vi "play_AFMss_integral_trajTrack.vi"() -> ()   [LabVIEW 2017]
uses:
  controls/controlParams_tracktraj.ctl
  <vilib>/userdefined/High Color/nirio_resource_hc.ctl
  <vilib>/Utility/file.llb/Read From Spreadsheet File (DBL).vi
  <vilib>/FPGAPlugInAG/cRIO-9082/niLvFpga_Open_cRIO-9082.vi
  <vilib>/rvi/interface/common/dynamic/niFpgaDynamicAddResources.vi
  <vilib>/FPGAPlugInAG/Dynamic/niLvFpga_Reset_Dynamic.vi
  <vilib>/rvi/interface/common/niFpgaWaitOnOcc.vi
  <vilib>/Utility/error.llb/Error Cluster From Error Code.vi
  <vilib>/rvi/errors/niLvFpgaAdjustHostInterfaceError.vi
  <vilib>/FPGAPlugInAG/Dynamic/niLvFpga_Run_Dynamic.vi
  <vilib>/Utility/file.llb/Write To Spreadsheet File (DBL).vi
  <vilib>/FPGAPlugInAG/Dynamic/niLvFpga_Close_Dynamic.vi
  <vilib>/rvi/interface/nirviOpenFPGA/nirviOpenFPGA.xnode
  FPGA Bitfiles/AFMsssinglematri_FPGATargetSPARTA_AFMsscontrolDela_bcNq5xaO9wQ.lvbitx
  <vilib>/rvi/interface/nirviMethod/nirviMethod.xnode
  <vilib>/rvi/interface/nirviReadWriteControl/nirviReadWriteControl.xnode
  <vilib>/rvi/interface/nirviCloseFPGA/nirviCloseFPGA.xnode
  <vilib>/FPGAPlugInAG/Dynamic/niLvFpga_ConfigureFifo_Dynamic.vi
  <vilib>/rvi/errors/niLvFpgaMergeErrorWithErrorCode.vi
  <vilib>/rvi/interface/Simulation/niFpgaSimulationCallBeginRW.vi
  <vilib>/FPGAPlugInAG/Dynamic/niLvFpga_ReadFifo_Dynamic.vi
  <vilib>/FPGAPlugInAG/Dynamic/niLvFpga_WriteFifo_Dynamic.vi
  NiFpgaLv.dll
panel:
  in  "control_data_path":path=path "C:/Users/arnold/Documents/MATLAB/AFM_SS/data/ref_traj_track.csv"
  out "Actual Depth":u32
  out "YK TO":bool
  out "UK TO":bool
  out "yk":sgl
  out "loop ticks benchmark":sgl
  out "Xd_out(k+1)":sgl[](array[numeric])
  in  "Cluster":T1={"umax"=3.0, "y_ref(k)"=0.0, "Ki"=0.0, "y(k) (from plant)"=0.0, "ND"=0, "NS"=0, "u_Kx_ref(k)"=0.0} {"u_Kx_ref(k)" format="%#_13g"; "Ki" format="%#_13g"; "y_ref(k)" format="%#_13g"; "umax" format="%#_13g"}
  out "Unstable Traj":bool
  out "Control Loop Done":bool
  out "Elements Remaining":u32
  out "Arow10":sgl[](array[numeric])=[0.0, 0.0, 0.0, 0.0, 0.0, 0.0, 0.90156674, 0.0, 0.0]
  out "Arow9":sgl[](array[numeric])=[0.0, 0.0, 0.0, 0.0, 0.0, 0.0, 0.90156674, 0.0, 0.0]
  out "Arow8":sgl[](array[numeric])=[0.0, 0.0, 0.0, 0.0, 0.0, 0.0, 0.90156674, 0.0, 0.0]
  out "elements left":i32=1
  in  "reference traj path":path=path "C:/Users/arnold/Documents/MATLAB/AFM_SS/data/ref_traj_track.csv"
  in  "outputData BOTH":path=path "C:/Users/arnold/Documents/MATLAB/AFM_SS/data/exp01outputBOTH.csv"
  out "x+1":i32
  out "ND":i32
  out "NS":i32
  in  "Tab Control":enum32{"Custom Params", "Loaded Params"}(tab)
  in  "Nbar":dbl=1.253469179440319 format="%#_13g"
  in  "Ki":dbl=0.125346917944 format="%#_13g"
  out "Nbar":dbl=1.253469179440319 format="%#_13g"
  out "Ki":dbl=0.125346917944 format="%#_13g"
  out "ref":dbl format="%#_13g"
  in  "SettleTicks":i32=10
  in  "Stop":bool=TRUE
  out "y iter":i32
  out "u iter":i32
  out "size(s) 5":i32
  out "size(s)":i32
  out "Arow7":sgl[](array[numeric])=[0.0, 0.0, 0.0, 0.0, 0.0, 0.0, 0.90156674, 0.0, 0.0]
  out "Arow6":sgl[](array[numeric])=[0.0, 0.0, 0.0, 0.0, -0.0009308535, 0.009943728, 1.1488396, 0.0, 0.0]
  out "Arow5":sgl[](array[numeric])=[0.0, 0.0, 0.0, 0.0, 0.99437284, 0.09308535, 3.730764, 0.0, 0.0]
  out "Arow4":sgl[](array[numeric])=[0.0, 0.0, -0.16696692, 0.97962993, 29.579603, 1.2871753, 39.36298, 0.0, 0.0]
  out "Arow3":sgl[](array[numeric])=[0.0, 0.0, 0.97962993, 0.16696692, 2.4679432, 0.11174757, 2.9240768, 0.0, 0.0]
  out "K_in 2":sgl[](array[numeric])=[-0.023819132, 0.00010408472, 0.0, 0.0, 0.0, 0.0, 0.0, 0.0, 0.0]
  out "K_in":sgl[](array[numeric])=[-0.023819132, 0.00010408472, 0.0, 0.0, 0.0, 0.0, 0.0, 0.0, 0.0]
  out "Arow2_in":sgl[](array[numeric])=[-0.21879435, 0.97156703, 5.4823804, 0.59487915, 7.8694544, 0.30187303, 8.202156, 0.0, 0.0]
  out "Arow1_in":sgl[](array[numeric])=[0.97156703, 0.21879435, 0.7281903, 0.07828272, 1.117765, 0.037789278, 0.6448556, 0.0, 0.0]
  out "C_in":sgl[](array[numeric])=[-8.076578e-08, -5.6617e-09, 2.3556278e-05, -6.9169624e-07, -0.005420799, 0.00037984832, -0.012524399, 0.0, 0.0]
  out "L_in":sgl[](array[numeric])=[-2254.4756, -17288.861, -3886.0125, -24956.67, -705.887, -3987.6506, -7.2153935, 0.0, 0.0]
  out "Bz_in":sgl[](array[numeric])=[-0.0016434871, -0.020676594, -0.010679029, -0.20639984, -0.030792456, -1.3413852, -0.02736353, 0.0, 0.0]
  in  "Iters":i32=25
  in  "Cont Run (F)":bool=TRUE
  in  "ymax":dbl=4.0 format="%#_13g"
  in  "umax":dbl=1.0 format="%#_13g"
  in  "TsTicks":i32=1600
  # "Manually define Parameters"
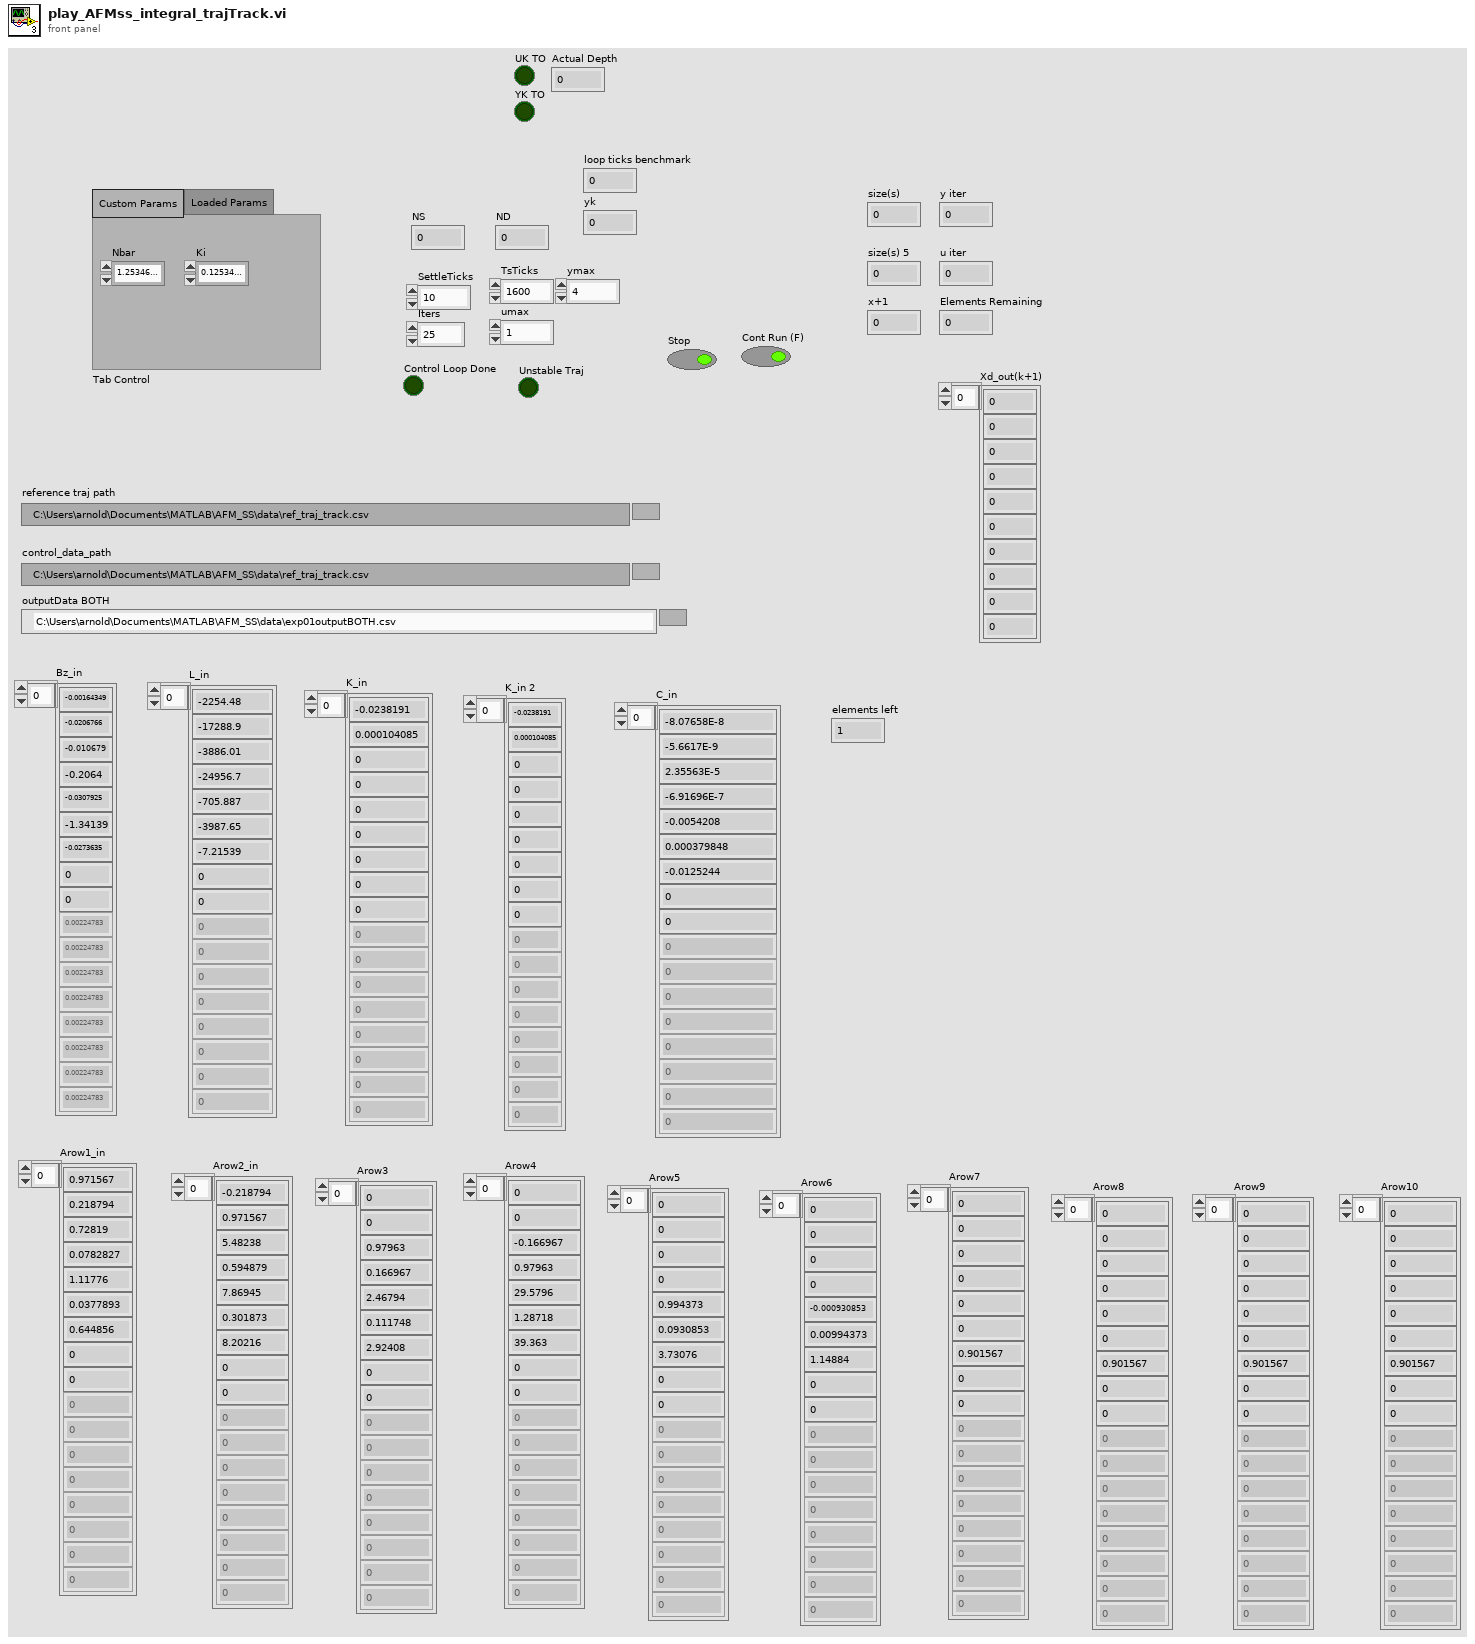
[diagram p1: front panel]
types:
  T1 = typedef "controlParams_tracktraj.ctl" = cluster{"umax":sgl, "y_ref(k)":sgl, "Ki":sgl, "y(k) (from plant)":sgl, "ND":i16, "NS":i16, "u_Kx_ref(k)":sgl}
  T2 = typedef "nirio_resource_hc.ctl" = tag
  T3 = typedef "ControlParams.ctl" = cluster{"NS":i32, "ND":i32, "Nbar":dbl, "Ki":dbl, "ref":dbl}
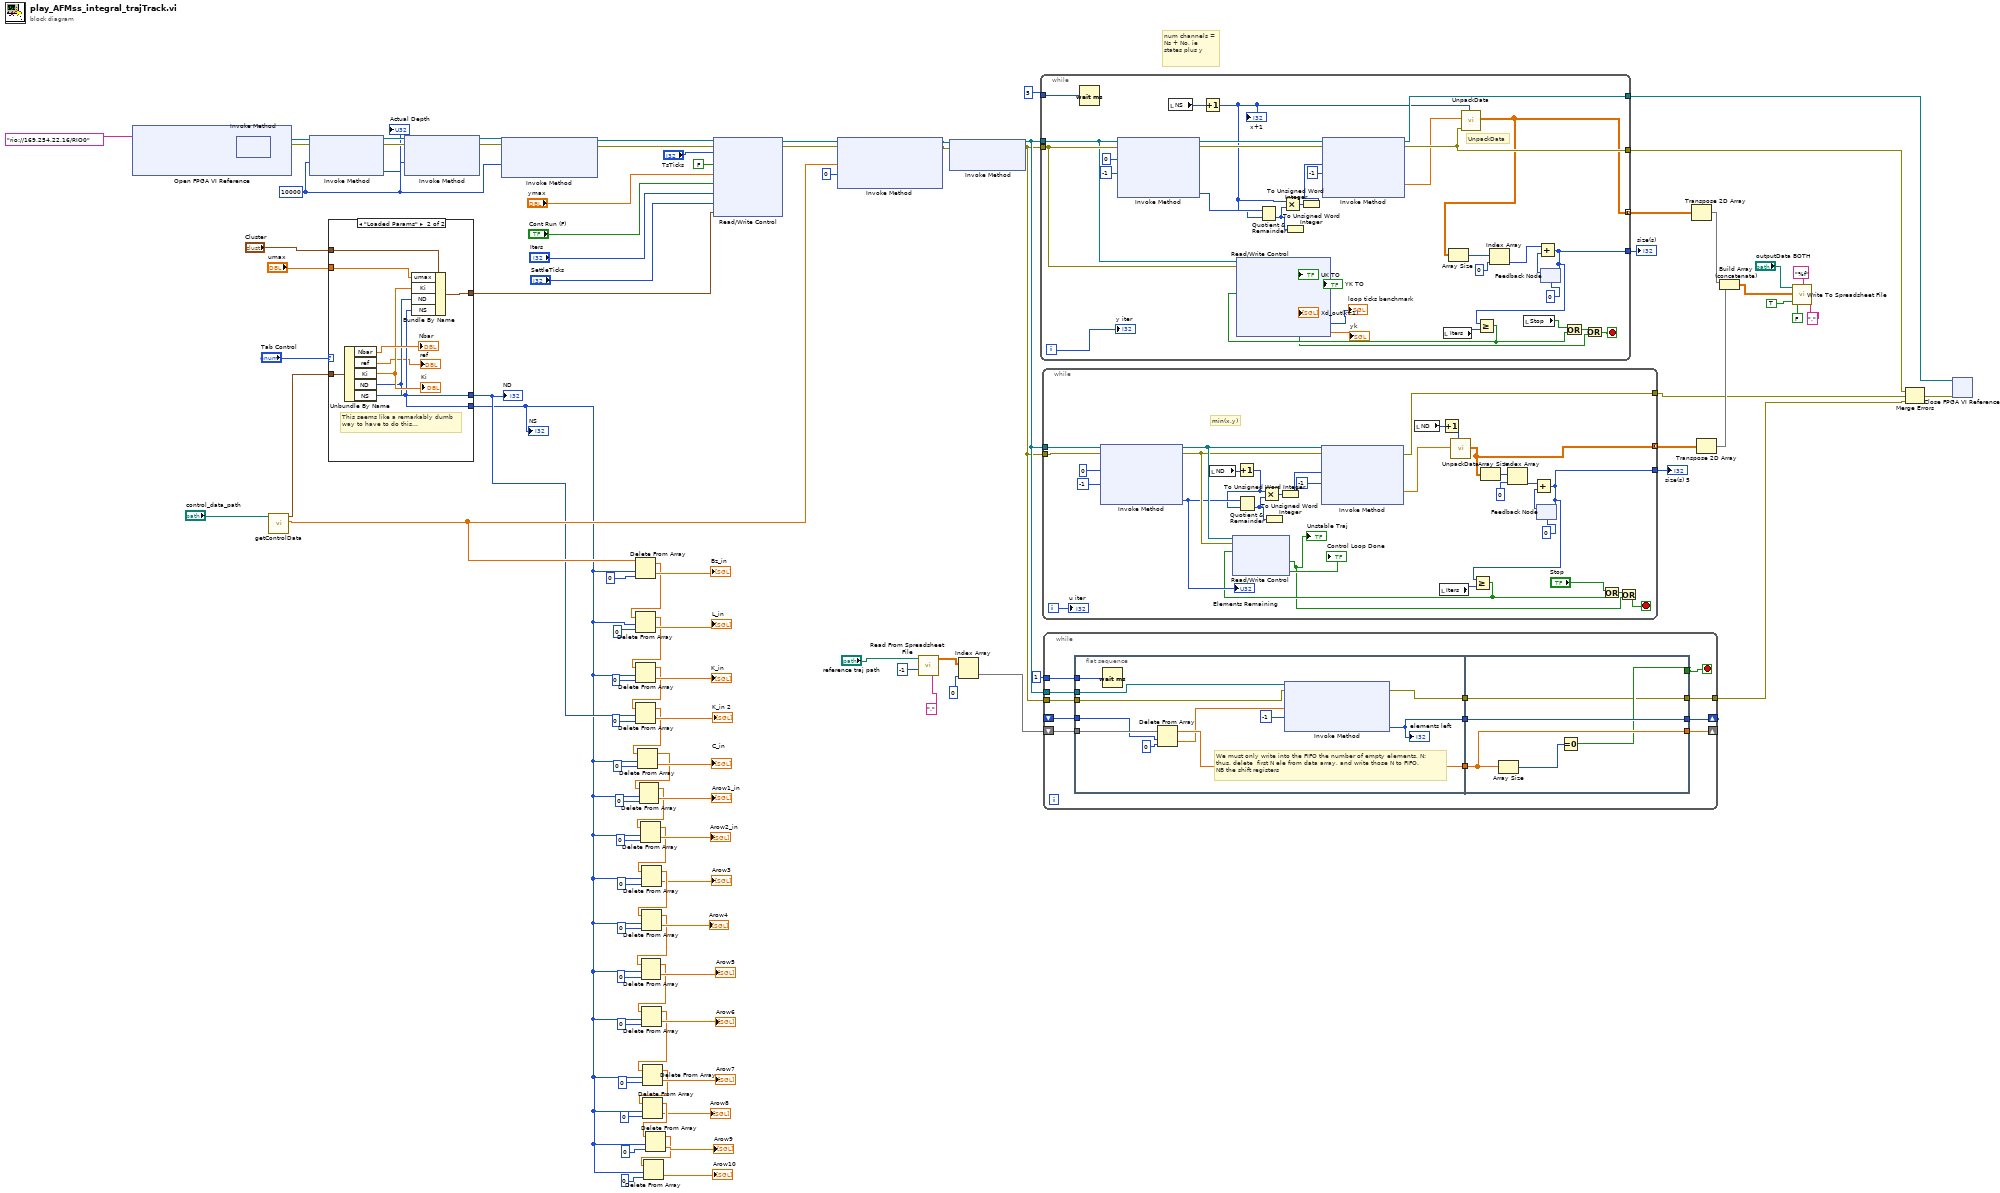
[diagram p0: block diagram]
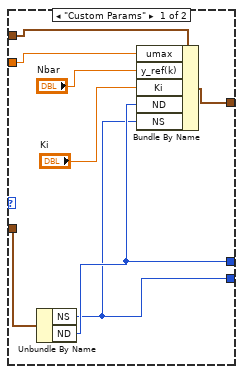
[diagram p2: hidden frame]
diagram:
  w45 = 10000
  # "num channels = Ns + No, ie states plus y"
  n1 = xnode "Open FPGA VI Reference"("resource name"=T2 "rio://169.254.22.16/RIO0") -> ("FPGA VI Reference Out"=w40:refnum<k20>, "error out"=w39:errorcluster)  [unwired: 1 in]
  n2 = xnode "Invoke Method"("FPGA VI Reference In"=w40, "error in"=w39) -> ("FPGA VI Reference Out"=w52:refnum<k20>, "error out"=w51:errorcluster)
  n3 = call "getControlData.vi"("system matricec path"="control_data_path") -> ("AllMatrix"=w44:dbl[], "controlParams"=w43:T3)  [unwired: 9 in]
  n4 = xnode "Invoke Method"("FPGA VI Reference In"=w52, "error in"=w51, "Requested Depth"=w45) -> ("FPGA VI Reference Out"=w104:refnum<k20>, "error out"=w103:errorcluster, "Actual Depth"=→"Actual Depth":u32)
  n5 = case shown="\"Loaded Params\"" "Tab Control" {
    tunnel: w43 -> [w112 w121]
    tunnel: [w106 w116] -> w10
    tunnel: [w107 w117] -> w41
    tunnel: "umax" -> [w111 w114]
    tunnel: [w109 w118] -> w7
    tunnel: "Cluster" -> [w105 w115]
    frame "Custom Params" {
      n6 = Unbundle By Name(w112) -> ("NS"=w106:i32, "ND"=w107:i32)
      n7 = Bundle By Name(cluster=w105, "umax"=w111, "y_ref(k)"="Nbar", "Ki"="Ki", "ND"=w107, "NS"=w106) -> (w109:T1)
    }
    frame "Loaded Params" {
      # "This seems like a remarkably dumb\nway to have to do this..."
      n8 = Unbundle By Name(w121) -> ("Nbar"=→"Nbar":dbl, "ref"=→"ref":dbl, "Ki"=w119:dbl, "ND"=w117:i32, "NS"=w116:i32)
      "Ki" <- w119
      n9 = Bundle By Name(cluster=w115, "umax"=w114, "Ki"=w119, "ND"=w117, "NS"=w116) -> (w118:T1)
    }
  }
  "NS" <- w10
  "ND" <- w41
  n10 = xnode "Invoke Method"("FPGA VI Reference In"=w104, "error in"=w103, "Requested Depth"=w45) -> ("FPGA VI Reference Out"=w49:refnum<k20>, "error out"=w48:errorcluster)  [unwired: 1 out]
  n11 = xnode "Invoke Method"("FPGA VI Reference In"=w49, "error in"=w48, "Requested Depth"=w45) -> ("FPGA VI Reference Out"=w47:refnum<k20>, "error out"=w46:errorcluster)  [unwired: 1 out]
  n12 = Delete From Array(array=w44, length=w10, index=0) -> (deleted portion=→"Bz_in":dbl[], array with subset deleted=w88:dbl[])
  n13 = Delete From Array(array=w88, length=w10, index=0) -> (deleted portion=→"L_in":dbl[], array with subset deleted=w85:dbl[])
  n14 = Delete From Array(array=w85, length=w10, index=0) -> (deleted portion=→"K_in":dbl[], array with subset deleted=w81:dbl[])
  n15 = Delete From Array(array=w81, length=w41, index=0) -> (deleted portion=→"K_in 2":dbl[], array with subset deleted=w78:dbl[])
  n16 = Delete From Array(array=w78, length=w10, index=0) -> (deleted portion=→"C_in":dbl[], array with subset deleted=w75:dbl[])
  n17 = Delete From Array(array=w75, length=w10, index=0) -> (deleted portion=→"Arow1_in":dbl[], array with subset deleted=w72:dbl[])
  n18 = Delete From Array(array=w72, length=w10, index=0) -> (deleted portion=→"Arow2_in":dbl[], array with subset deleted=w65:dbl[])
  n19 = Delete From Array(array=w65, length=w10, index=0) -> (deleted portion=→"Arow3":dbl[], array with subset deleted=w64:dbl[])
  n20 = Delete From Array(array=w64, length=w10, index=0) -> (deleted portion=→"Arow4":dbl[], array with subset deleted=w61:dbl[])
  n21 = Delete From Array(array=w61, length=w10, index=0) -> (deleted portion=→"Arow5":dbl[], array with subset deleted=w59:dbl[])
  n22 = Delete From Array(array=w59, length=w10, index=0) -> (deleted portion=→"Arow6":dbl[], array with subset deleted=w57:dbl[])
  n23 = Delete From Array(array=w57, length=w10, index=0) -> (deleted portion=→"Arow7":dbl[], array with subset deleted=w17:dbl[])
  n24 = Delete From Array(array=w17, length=w10, index=0) -> (deleted portion=→"Arow8":dbl[], array with subset deleted=w15:dbl[])
  n25 = Delete From Array(array=w15, length=w10, index=0) -> (deleted portion=→"Arow9":dbl[], array with subset deleted=w11:dbl[])
  n26 = Delete From Array(array=w11, length=w10, index=0) -> (deleted portion=→"Arow10":dbl[])  [unwired: 1 out]
  n27 = xnode "Read/Write Control"("FPGA VI Reference In"=w47, "error in"=w46, "TsTicks"="TsTicks", "Abort"=FALSE, "ymax"="ymax", "False  = cont run"="Cont Run (F)", "iters"="Iters", "Settle Ticks"="SettleTicks", "Cluster"=w7) -> ("FPGA VI Reference Out"=w93:refnum<k20>, "error out"=w92:errorcluster)
  n28 = xnode "Invoke Method"("FPGA VI Reference In"=w93, "error in"=w92, "Data"=w44, "Timeout (ms)"=0) -> ("FPGA VI Reference Out"=w96:refnum<k20>, "error out"=w95:errorcluster)  [unwired: 1 out]
  n29 = call-poly <vilib>:"Read From Spreadsheet File.vi"("delimiter (\\t)"=",", "number of rows (all:-1)"=-1, "file path (dialog if empty)"="reference traj path") -> ("all rows"=w24:dbl[][])  [unwired: 4 in, 4 out]
  n30 = xnode "Invoke Method"("FPGA VI Reference In"=w96, "error in"=w95) -> ("FPGA VI Reference Out"=w5:refnum<k20>, "error out"=w4:errorcluster)  [unwired: 1 in]
  n31 = Index Array(array=w24, index (col)=0 ("dimension size")) -> (element=w22:dbl[])  [unwired: 1 in]
  n32 = while {
    tunnel: 5 -> [w157]
    tunnel: w5 -> [w135]
    tunnel: w4 -> [w136]
    tunnel: [w149] -> w21
    tunnel: [w148] -> w91
    tunnel: [w134] -> w55 mode=concatenating
    tunnel: [w132] -> w53
    i -> [w133]
    stop <- w127 stop-if-true
    # "UnpackData"
    n33 = Wait (ms)(milliseconds to wait=w157) -> ()  [unwired: 1 out]
    n34 = xnode "Invoke Method"("FPGA VI Reference In"=w135, "error in"=w136, "Number of Elements"=0 ("Timeout (ms)"), "Timeout (ms)"=-1) -> ("FPGA VI Reference Out"=w153:refnum<k20>, "error out"=w154:errorcluster, "Elements Remaining"=w144:u32)  [unwired: 1 out]
    n35 = local read "NS"() -> (w143:i32)
    n36 = Increment(x=w143) -> (x+1=w142:i32)
    "x+1" <- w142
    n37 = Quotient & Remainder(x=w144, y=w142) -> (floor(x/y)=w146:u32)  [unwired: 1 out]
    n38 = Multiply(x=w142, y=w146) -> (x*y=w151:u32)
    n39 = To Unsigned Word Integer(number=w146) -> ()  [unwired: 1 out]
    n40 = To Unsigned Word Integer(number=w151) -> (unsigned 16bit integer=w147:u16)
    n41 = xnode "Invoke Method"("FPGA VI Reference In"=w153, "error in"=w154, "Number of Elements"=w147, "Timeout (ms)"=-1) -> ("FPGA VI Reference Out"=w148:refnum<k20>, "error out"=w149:errorcluster, "Data"=w141:sgl[])  [unwired: 1 out]
    n42 = local read "Iters"() -> (w145:i32)
    n43 = call "UnpackData.vi"("NumChannels"=w142, "error In"=w149, "1D Data In"=w141) -> ("2D Data Out"=w134:dbl[][])  [unwired: 7 in, 1 out]
    n44 = Array Size(array=w134) -> (size(s)=w140:i32[])
    n45 = Index Array(array=w140, index=0) -> (element=w138:i32)
    n46 = local read "Stop"() -> (w130:bool)
    n47 = feedback #1(0) -> (w139:i32)
    n48 = Add(x=w138, y=w139) -> (x+y=w132:i32)
    n49 = Greater Or Equal?(x=w132, y=w145) -> (x >= y?=w131:bool)
    n50 = xnode "Read/Write Control"("FPGA VI Reference In"=w135, "error in"=w136, "Abort"=w131) -> ("UK TO"=→"UK TO":bool, "YK TO"=→"YK TO":bool, "Unstable Traj"=w128:bool, "Xd_out(k+1)"=→"Xd_out(k+1)":sgl[], "Loop Ticks (benchmark)"=→"loop ticks benchmark":i16, "yk"=→"yk":sgl)  [unwired: 2 out]
    n51 = feedback-in #1(w132) -> ()
    n52 = Or(x=w130, y=w131) -> (x .or. y?=w129:bool)
    n53 = Or(x=w129, y=w128) -> (x .or. y?=w127:bool)
    "y iter" <- w133
  }
  "size(s)" <- w53
  n54 = while {
    tunnel: [w166] -> w42 mode=concatenating
    tunnel: w5 -> [w176]
    tunnel: w4 -> [w175]
    tunnel: [w173] -> w54
    tunnel: [w162] -> w19
    i -> [w174]
    stop <- w161 stop-if-true
    # "min(x,y)"
    n55 = xnode "Invoke Method"("FPGA VI Reference In"=w176, "error in"=w175, "Number of Elements"=0 ("Timeout (ms)"), "Timeout (ms)"=-1) -> ("FPGA VI Reference Out"=w184:refnum<k20>, "error out"=w183:errorcluster, "Elements Remaining"=w180:u32)  [unwired: 1 out]
    "Elements Remaining" <- w180
    n56 = local read "ND"() -> (w169:i32)
    n57 = Increment(x=w169) -> (x+1=w178:i32)
    n58 = Quotient & Remainder(x=w180, y=w178) -> (floor(x/y)=w181:u32)  [unwired: 1 out]
    n59 = Multiply(x=w178, y=w181) -> (x*y=w182:u32)
    n60 = To Unsigned Word Integer(number=w181) -> ()  [unwired: 1 out]
    n61 = To Unsigned Word Integer(number=w182) -> (unsigned 16bit integer=w179:u16)
    n62 = xnode "Invoke Method"("FPGA VI Reference In"=w184, "error in"=w183, "Number of Elements"=w179, "Timeout (ms)"=-1) -> ("error out"=w162:errorcluster, "Data"=w170:sgl[])  [unwired: 2 out]
    n63 = local read "ND"() -> (w168:i32)
    n64 = local read "Iters"() -> (w185:i32)
    n65 = Increment(x=w168) -> (x+1=w165:i32)
    n66 = call "UnpackData.vi"("NumChannels"=w165, "1D Data In"=w170) -> ("2D Data Out"=w166:dbl[][])  [unwired: 8 in, 1 out]
    n67 = Array Size(array=w166) -> (size(s)=w163:i32[])
    n68 = Index Array(array=w163, index=0) -> (element=w167:i32)
    n69 = feedback #2(0) -> (w177:i32)
    n70 = Add(x=w167, y=w177) -> (x+y=w173:i32)
    n71 = Greater Or Equal?(x=w173, y=w185) -> (x >= y?=w172:bool)
    n72 = xnode "Read/Write Control"("FPGA VI Reference In"=w184, "error in"=w183, "Abort"=w172) -> ("Unstable Traj"=w158:bool, "Loop Done"=→"Control Loop Done":bool)  [unwired: 2 out]
    "Unstable Traj" <- w158
    n73 = feedback-in #2(w173) -> ()
    n74 = Or(x="Stop", y=w172) -> (x .or. y?=w160:bool)
    n75 = Or(x=w160, y=w158) -> (x .or. y?=w161:bool)
    "u iter" <- w174
  }
  "size(s) 5" <- w54
  n76 = while {
    tunnel: [w199] -> w18
    tunnel: 1 -> [w201]
    shift-right: [w194] -> _
    shift-left: _ -> [w198]
    shift-right: [w192] -> _
    shift-left: w22 -> [w200]
    tunnel: w5 -> [w191]
    tunnel: w4 -> [w190]
    stop <- w195 stop-if-true
    n77 = flat-sequence {
      tunnel: w201 -> [w212]
      tunnel: w200 -> [w207]
      tunnel: w198 -> [w203]
      tunnel: [w210] -> w197
      tunnel: [w208] -> w196
      tunnel: [w209] -> w193
      tunnel: w191 -> [w205]
      tunnel: w190 -> [w204]
      tunnel: [w217] -> w194
      tunnel: [w213] -> w199
      tunnel: w197 -> [w213]
      tunnel: w196 -> [w217]
      tunnel: [w214] -> w195
      tunnel: w193 -> [w215]
      tunnel: [w215] -> w192
      frame #0 {
        # "We must only write into the FIFO the number of empty elements, N:\nthus, delete  first N ele from data array, and write those N to FIFO.\nNB the shift registers"
        n78 = Wait (ms)(milliseconds to wait=w212) -> ()  [unwired: 1 out]
        n79 = Delete From Array(array=w207, length=w203, index=0) -> (deleted portion=w206:dbl[], array with subset deleted=w209:dbl[])
        n80 = xnode "Invoke Method"("FPGA VI Reference In"=w205, "error in"=w204, "Data"=w206, "Timeout (ms)"=-1) -> ("error out"=w210:errorcluster, "Empty Elements Remaining"=w208:u32)  [unwired: 1 out]
        "elements left" <- w208
      }
      frame #1 {
        n81 = Array Size(array=w215) -> (size(s)=w216:i32)
        n82 = Equal To 0?(x=w216) -> (x = 0?=w214:bool)
      }
    }
  }
  n83 = Transpose 2D Array(2D array=w55) -> (transposed array=w36:dbl[][])
  n84 = Transpose 2D Array(2D array=w42) -> (transposed array=w35:dbl[][])
  n85 = Build Array (concatenate)(w36, w35) -> (w29:dbl[][])
  n86 = call-poly <vilib>:"Write To Spreadsheet File.vi"("delimiter (\\t)"=",", "transpose? (no:F)"=TRUE, "format (%.3f)"="%f", "append to file? (new file:F)"=FALSE, "2D data"=w29, "file path (dialog if empty)"="outputData BOTH") -> ()  [unwired: 2 in, 1 out]
  n87 = Merge Errors(w21, w19, w18) -> (w20:errorcluster)
  n88 = xnode "Close FPGA VI Reference"("FPGA VI Reference In"=w91, "error in"=w20) -> ()  [unwired: 1 out]
